vi "Harvest.vi"(1 "Y":dbl, 2 "X":dbl) -> ()   [LabVIEW 2014]
panel:
  in  "diff":dbl
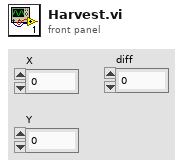
[diagram p1: front panel]
types:
  T1 = typedef "WPI_MotorControlDeviceRef.ctl" = cluster{"DeviceStatus":errorcluster, "Type":T2, "PWM":cluster{"Controller":T3, "PWM Channel":T4, "DeadBand":T5}, "CAN":cluster{"Device Number":u8, "Control Mode":T6, "Semaphore":T7, "Max Vout":dbl, "TalonSRX Control Mode":T8}, "Invert":bool, "TransformRef":T9, "InvTransformRef":T9}
  T2 = typedef "WPI_MotorControlType.ctl" = enum16{"PWM", "CAN", "CANTalonSRX"}
  T3 = typedef "FPGA_TypedefDigitalModule.ctl" = enum16{"Controller 1"}
  T4 = typedef "FPGA_DIOPWMChannel.ctl" = enum8{"PWM 0", "PWM 1", "PWM 2", "PWM 3", "PWM 4", "PWM 5", "PWM 6", "PWM 7", "PWM 8", "PWM 9", "PWM MXP 0", "PWM MXP 1", "PWM MXP 2", "PWM MXP 3", "PWM MXP 4", "PWM MXP 5", "PWM MXP 6", "PWM MXP 7", "PWM MXP 8", "PWM MXP 9", "Invalid"}
  T5 = typedef "WPI_PWMDeadband.ctl" = cluster{"Name":string, "maxPositivePwm":i32, "minPositivePwm":i32, "centerPwm":i32, "maxNegativePwm":i32, "minNegativePwm":i32, "angularRange":u16}
  T6 = typedef "WPI_CANJaguar_ControlMode.ctl" = enum8{"Percent VBus", "Current", "Speed", "Position", "Voltage"}
  T7 = typedef "Semaphore RefNum" = refnum<k1>
  T8 = typedef "WPI_CANTalonSRX_APIControlMode.ctl" = enum8{"Percent VBus", "Speed", "Position", "Slave", "Unchanged / Invalid"}
  T9 = typedef "WPI_PWMTransform_ConPane.ctl" = refnum<vi>
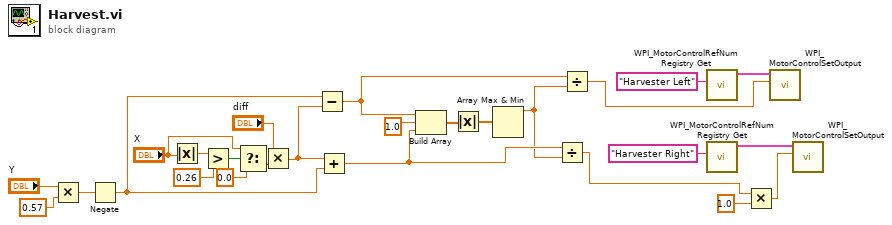
[diagram p0: block diagram]
diagram:
  n1 = Multiply(x="Y", y=0.57) -> (x*y=w2:dbl)
  n2 = Negate(x=w2) -> (-x=w21:dbl)
  n3 = Absolute Value(x="X") -> (abs(x)=w9:dbl)
  n4 = Greater?(x=w9, y=0.26) -> (0:w7:bool)
  n5 = Select(t="X", s=w7, f=0.0) -> (s? t:f=w6:dbl)
  n6 = Multiply(x="diff", y=w6) -> (x*y=w20:dbl)
  n7 = Subtract(x=w21, y=w20) -> (x-y=w13:dbl)
  n8 = Add(x=w20, y=w21) -> (x+y=w15:dbl)
  n9 = Build Array(w13, 1.0 ("element"), w15) -> (w17:dbl[])
  n10 = Absolute Value(x=w17) -> (abs(x)=w16:dbl[])
  n11 = Array Max & Min(array=w16) -> (max value=w14:dbl)  [unwired: 3 out]
  n12 = Divide(x=w15, y=w14) -> (x/y=w12:dbl)
  n13 = Divide(x=w13, y=w14) -> (x/y=w11:dbl)
  n14 = call <vilib>:"WPI_MotorControlRefNum Registry Get.vi"("refnum name"="Harvester Left") -> ("MotorControlDevRef"=w10:T1)  [unwired: 9 in, 1 out]
  n15 = call <vilib>:"WPI_MotorControlRefNum Registry Get.vi"("refnum name"="Harvester Right") -> ("MotorControlDevRef"=w25:T1)  [unwired: 9 in, 1 out]
  n16 = Multiply(x=w12, y=1.0) -> (x*y=w22:dbl)
  n17 = call <vilib>:"WPI_MotorControlSetOutput.vi"("Output"=w11, "MotorControlDevRef"=w10) -> ()  [unwired: 7 in, 3 out]
  n18 = call <vilib>:"WPI_MotorControlSetOutput.vi"("Output"=w22, "MotorControlDevRef"=w25) -> ()  [unwired: 7 in, 3 out]
